vi "CHEM_BOX_TEST_APP.vi"() -> ()   [LabVIEW 2011]
uses:
  <vilib>/Instr/_visa.llb/VISA Set IO Buffer Mask.ctl
  <vilib>/Platform/TimedLoop/XDataNode/timing_clust.ctl
  <vilib>/Platform/TimedLoop/XDataNode/nitl_modes.ctl
  <vilib>/Platform/TimedLoop/XDataNode/wakeup.ctl
  <vilib>/Instr/_visa.llb/VISA Configure Serial Port (Instr).vi
  <vilib>/Platform/TimedLoop/XDataNode/XDataNode.xnode
  <vilib>/Platform/TimedLoop/XDataNode/XDNodeRunTimeDep.lvlib
panel:
  out "4 to 20mA Inputs":dbl[](array[numeric]) format="%#5_5g"
  in  "Stream Inputs":bool
  out "Temperature Sensors":dbl[](array[numeric]) format="%#1_2g"
  out "MISC ADC Inputs":dbl[](array[numeric]) format="%#1_3g"
  out "MFC ADC Inputs":dbl[](array[numeric]) format="%#3_3g"
  in  "MFC Power Control":bool
  in  "MISC DAC Outputs":dbl[](array[slide]) scale=0.0..5.0
  in  "MFC DAC Outputs":dbl[](array[slide])=[0.0, 0.0, 0.0, 0.0, 0.0, 0.0, 0.0] scale=0.0..5.0
  in  "Misc Digital Outputs":bool[](array[boolean])=[FALSE, FALSE, FALSE, FALSE]
  in  "Solenoid Channels":bool[](array[boolean])=[FALSE, FALSE, FALSE, FALSE, FALSE, FALSE, FALSE, FALSE, FALSE, FALSE, FALSE, FALSE]
  in  "FAN CONTROL":bool
  in  "Disable All Heaters and Solenoids":bool
  out "Output Commands":string
  in  "Heater Channels":bool[](array[boolean])=[FALSE, FALSE, FALSE, FALSE, FALSE, FALSE, FALSE, FALSE]
  in  "COM PORT":refnum<visa-resource-name>
  out "Output Command Queue":refnum<queue>
  in  "?":bool
  out "Input Command Queue":refnum<queue>
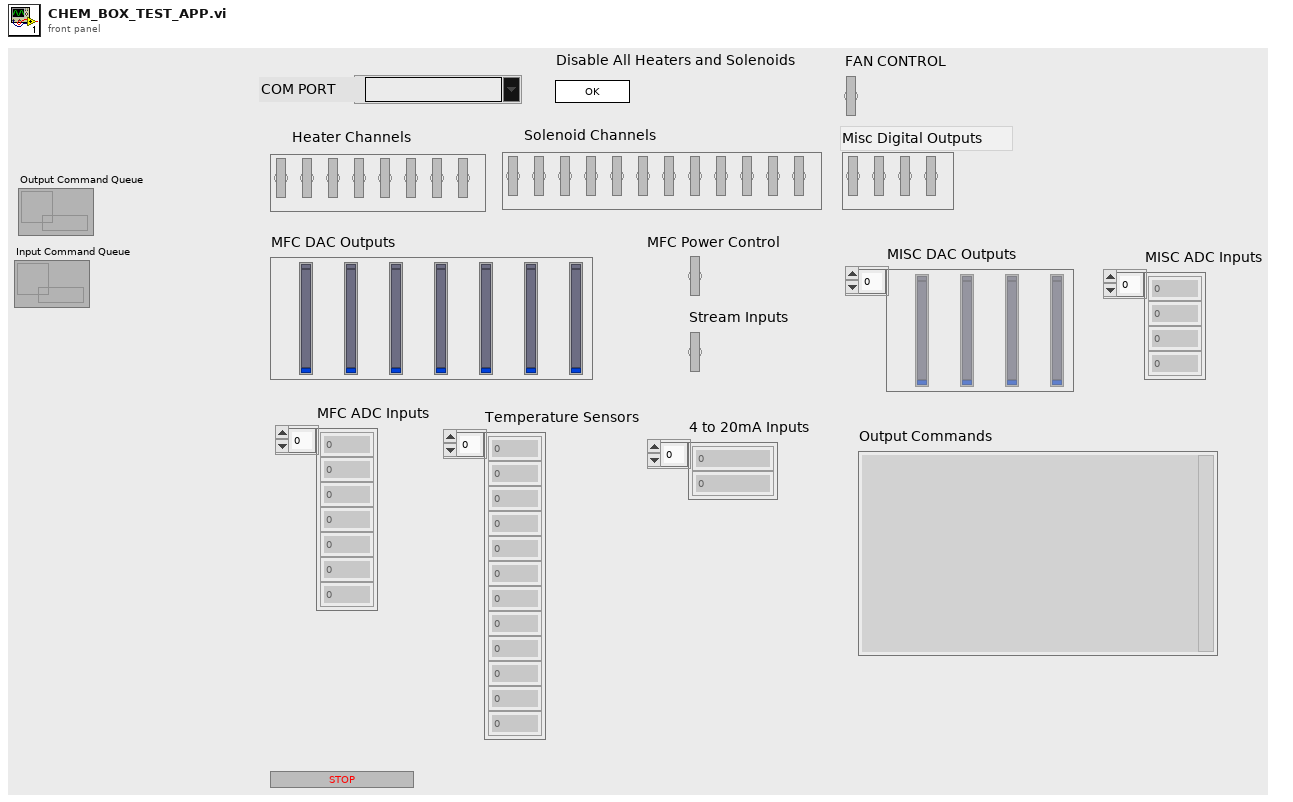
[diagram p1: front panel]
types:
  T1 = typedef "XDNodeRunTimeDep.lvlib/timing_clust.ctl" = cluster{"Expected End [f-1]":u64, "Actual End [f-1]":u64, "Finished Late? [f-1]":bool, "Expected End [i-1]":u64, "Actual End [i-1]":u64, "Finished Late? [i-1]":bool, "Expected Start [i]":u64, "Actual Start [i]":u64, "Expected Start [f]":u64, "Actual Start [f]":u64, "Source Name":string, "Structure Name":string, "Period":i64, "Deadline":i64, "Offset":i64, "Start":i64, "Priority":i32, "Timeout":i32, "Mode":T2, "Wakeup Reason":T3, "Error":errorcluster, "Source Type":string, "Secondary Source Type":string, "Global End Time":u64, "Global Start Time":u64, "Frame Duration":u64, "Iteration Duration":u64, "Assigned CPU":i32, "I/O Scan Engine Mode":u32}
  T2 = typedef "XDNodeRunTimeDep.lvlib/nitl_modes.ctl" = enum32{"No Change", "Process missed periods, maintain original phase", "Discard missed periods, maintain original phase", "Process missed periods, ignore original phase", "Discard missed periods, ignore original phase"}
  T3 = typedef "XDNodeRunTimeDep.lvlib/wakeup.ctl" = enum32{"Normal", "Aborted", "Asynchronous wakeup", "Timing source error", "Timed loop error", "Timeout"}
  T4 = typedef "VISA Set IO Buffer Mask.ctl" = u16
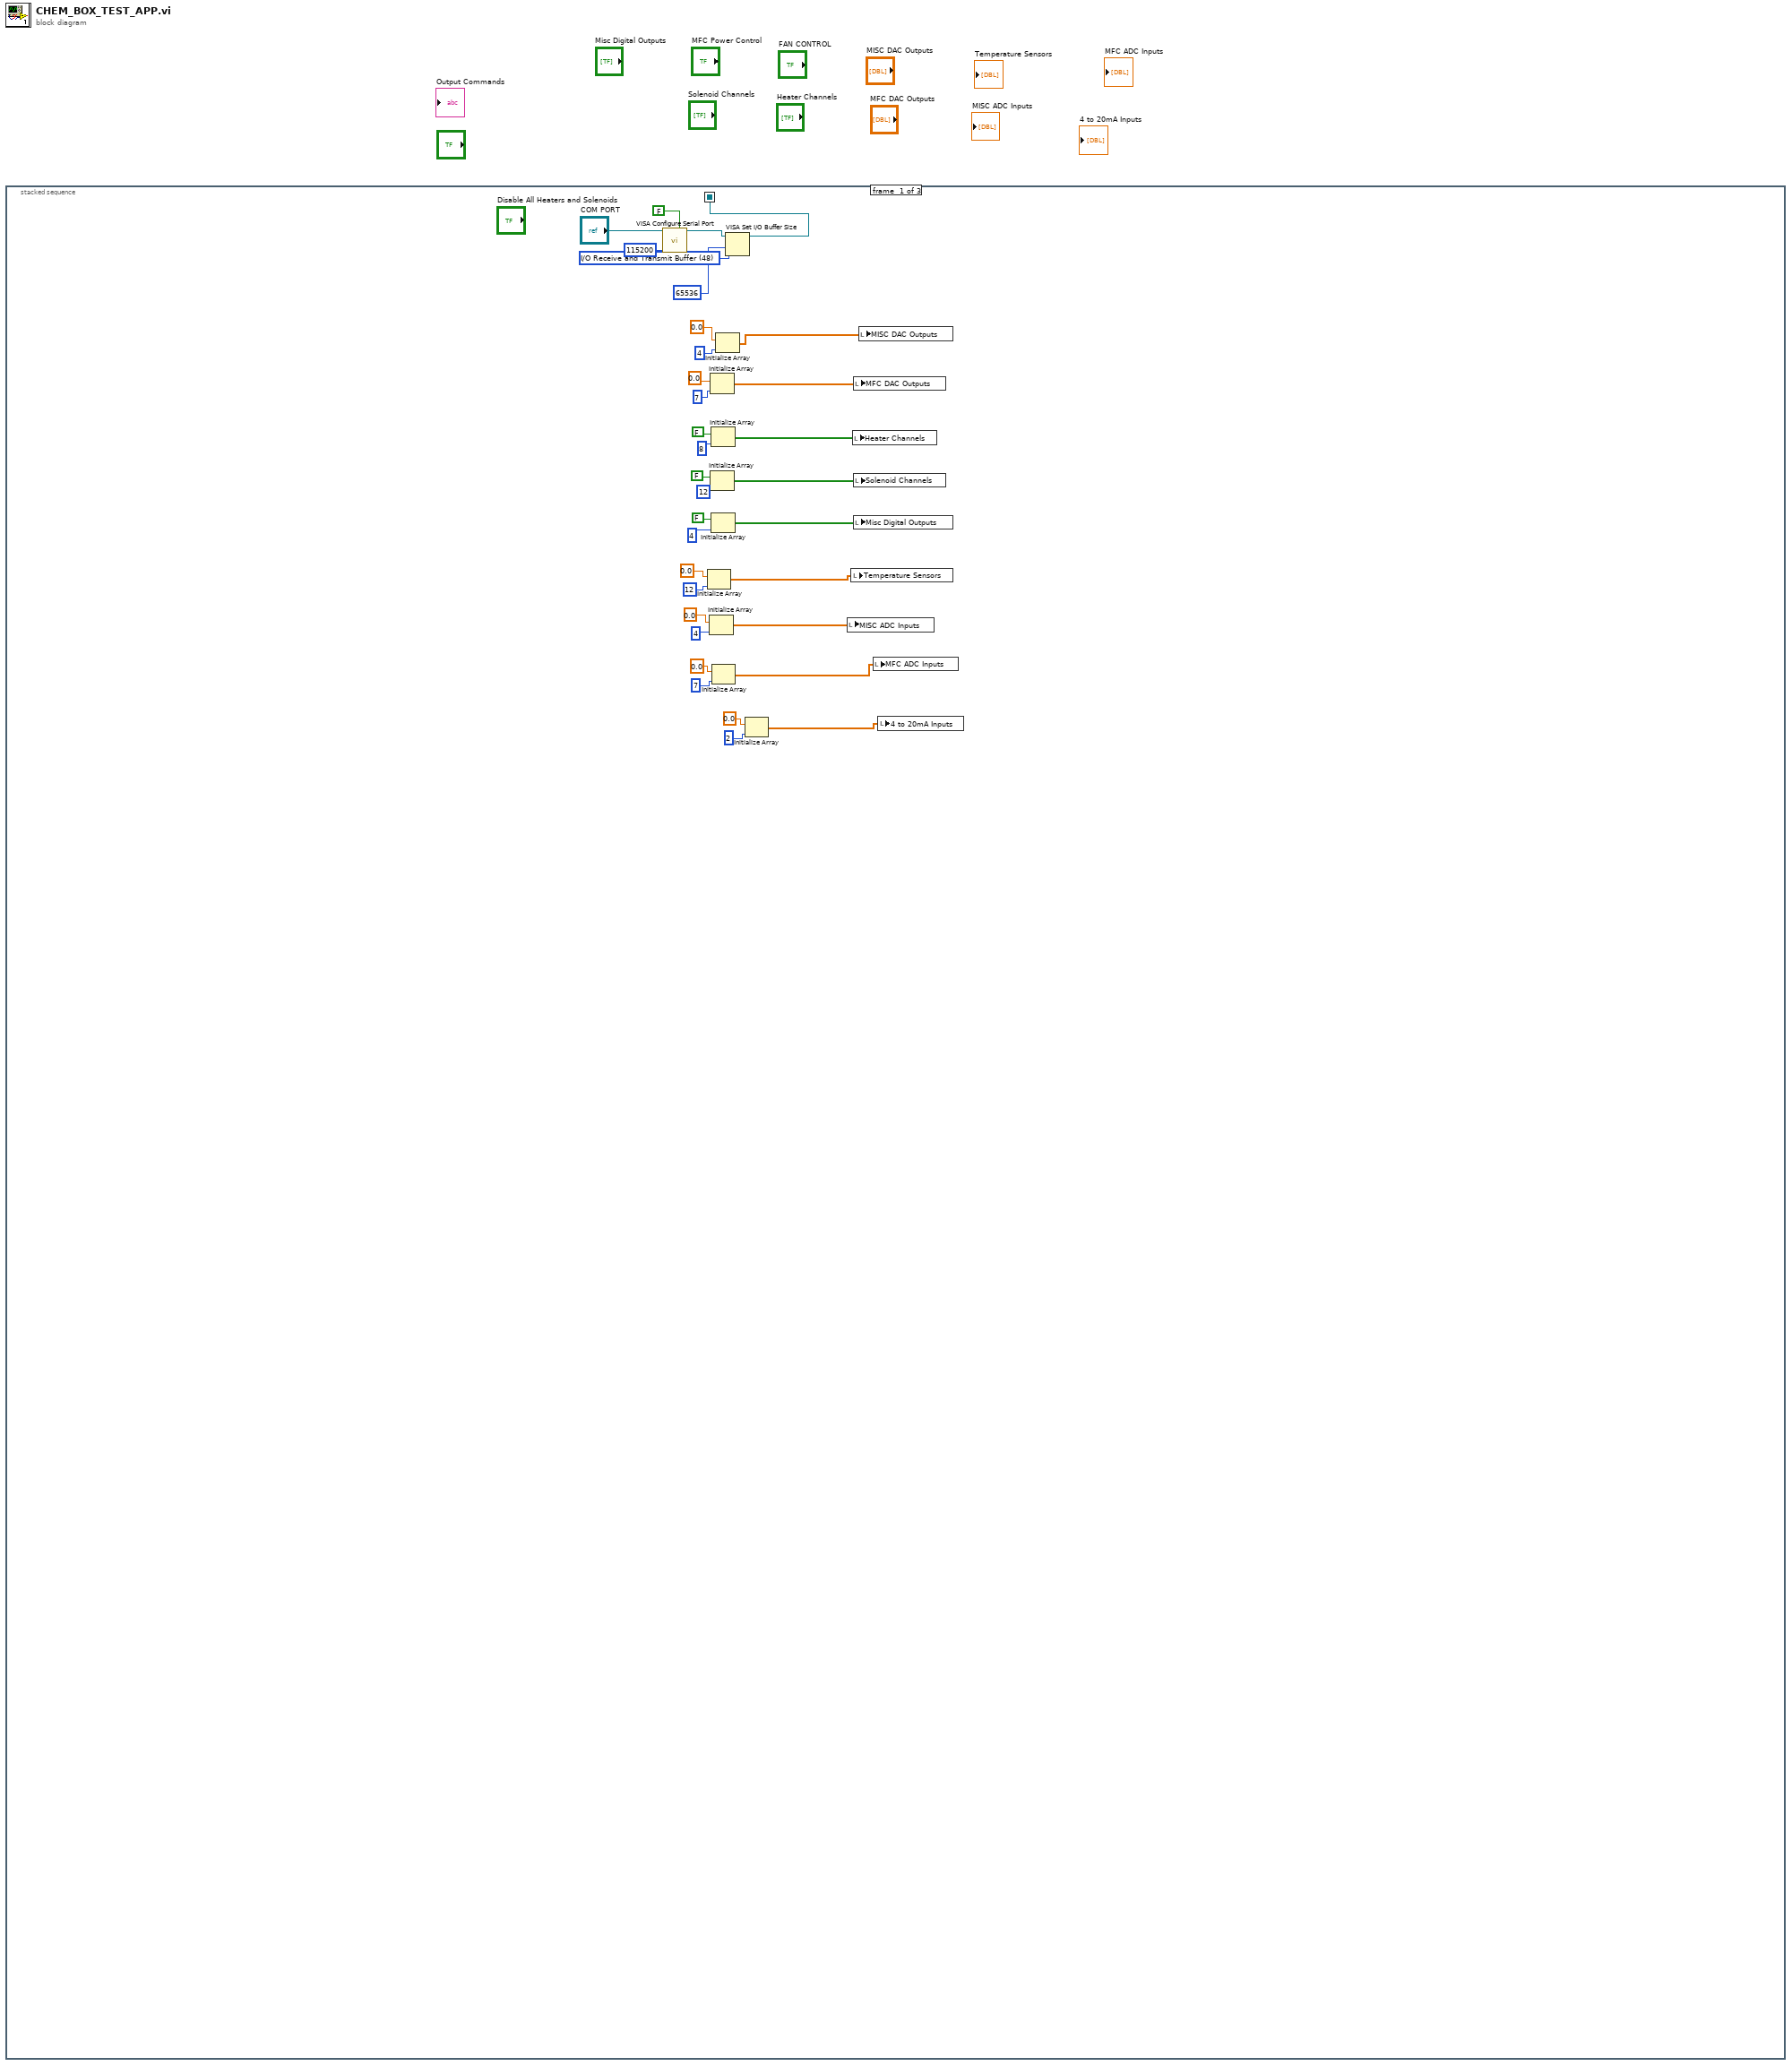
[diagram p0: block diagram]
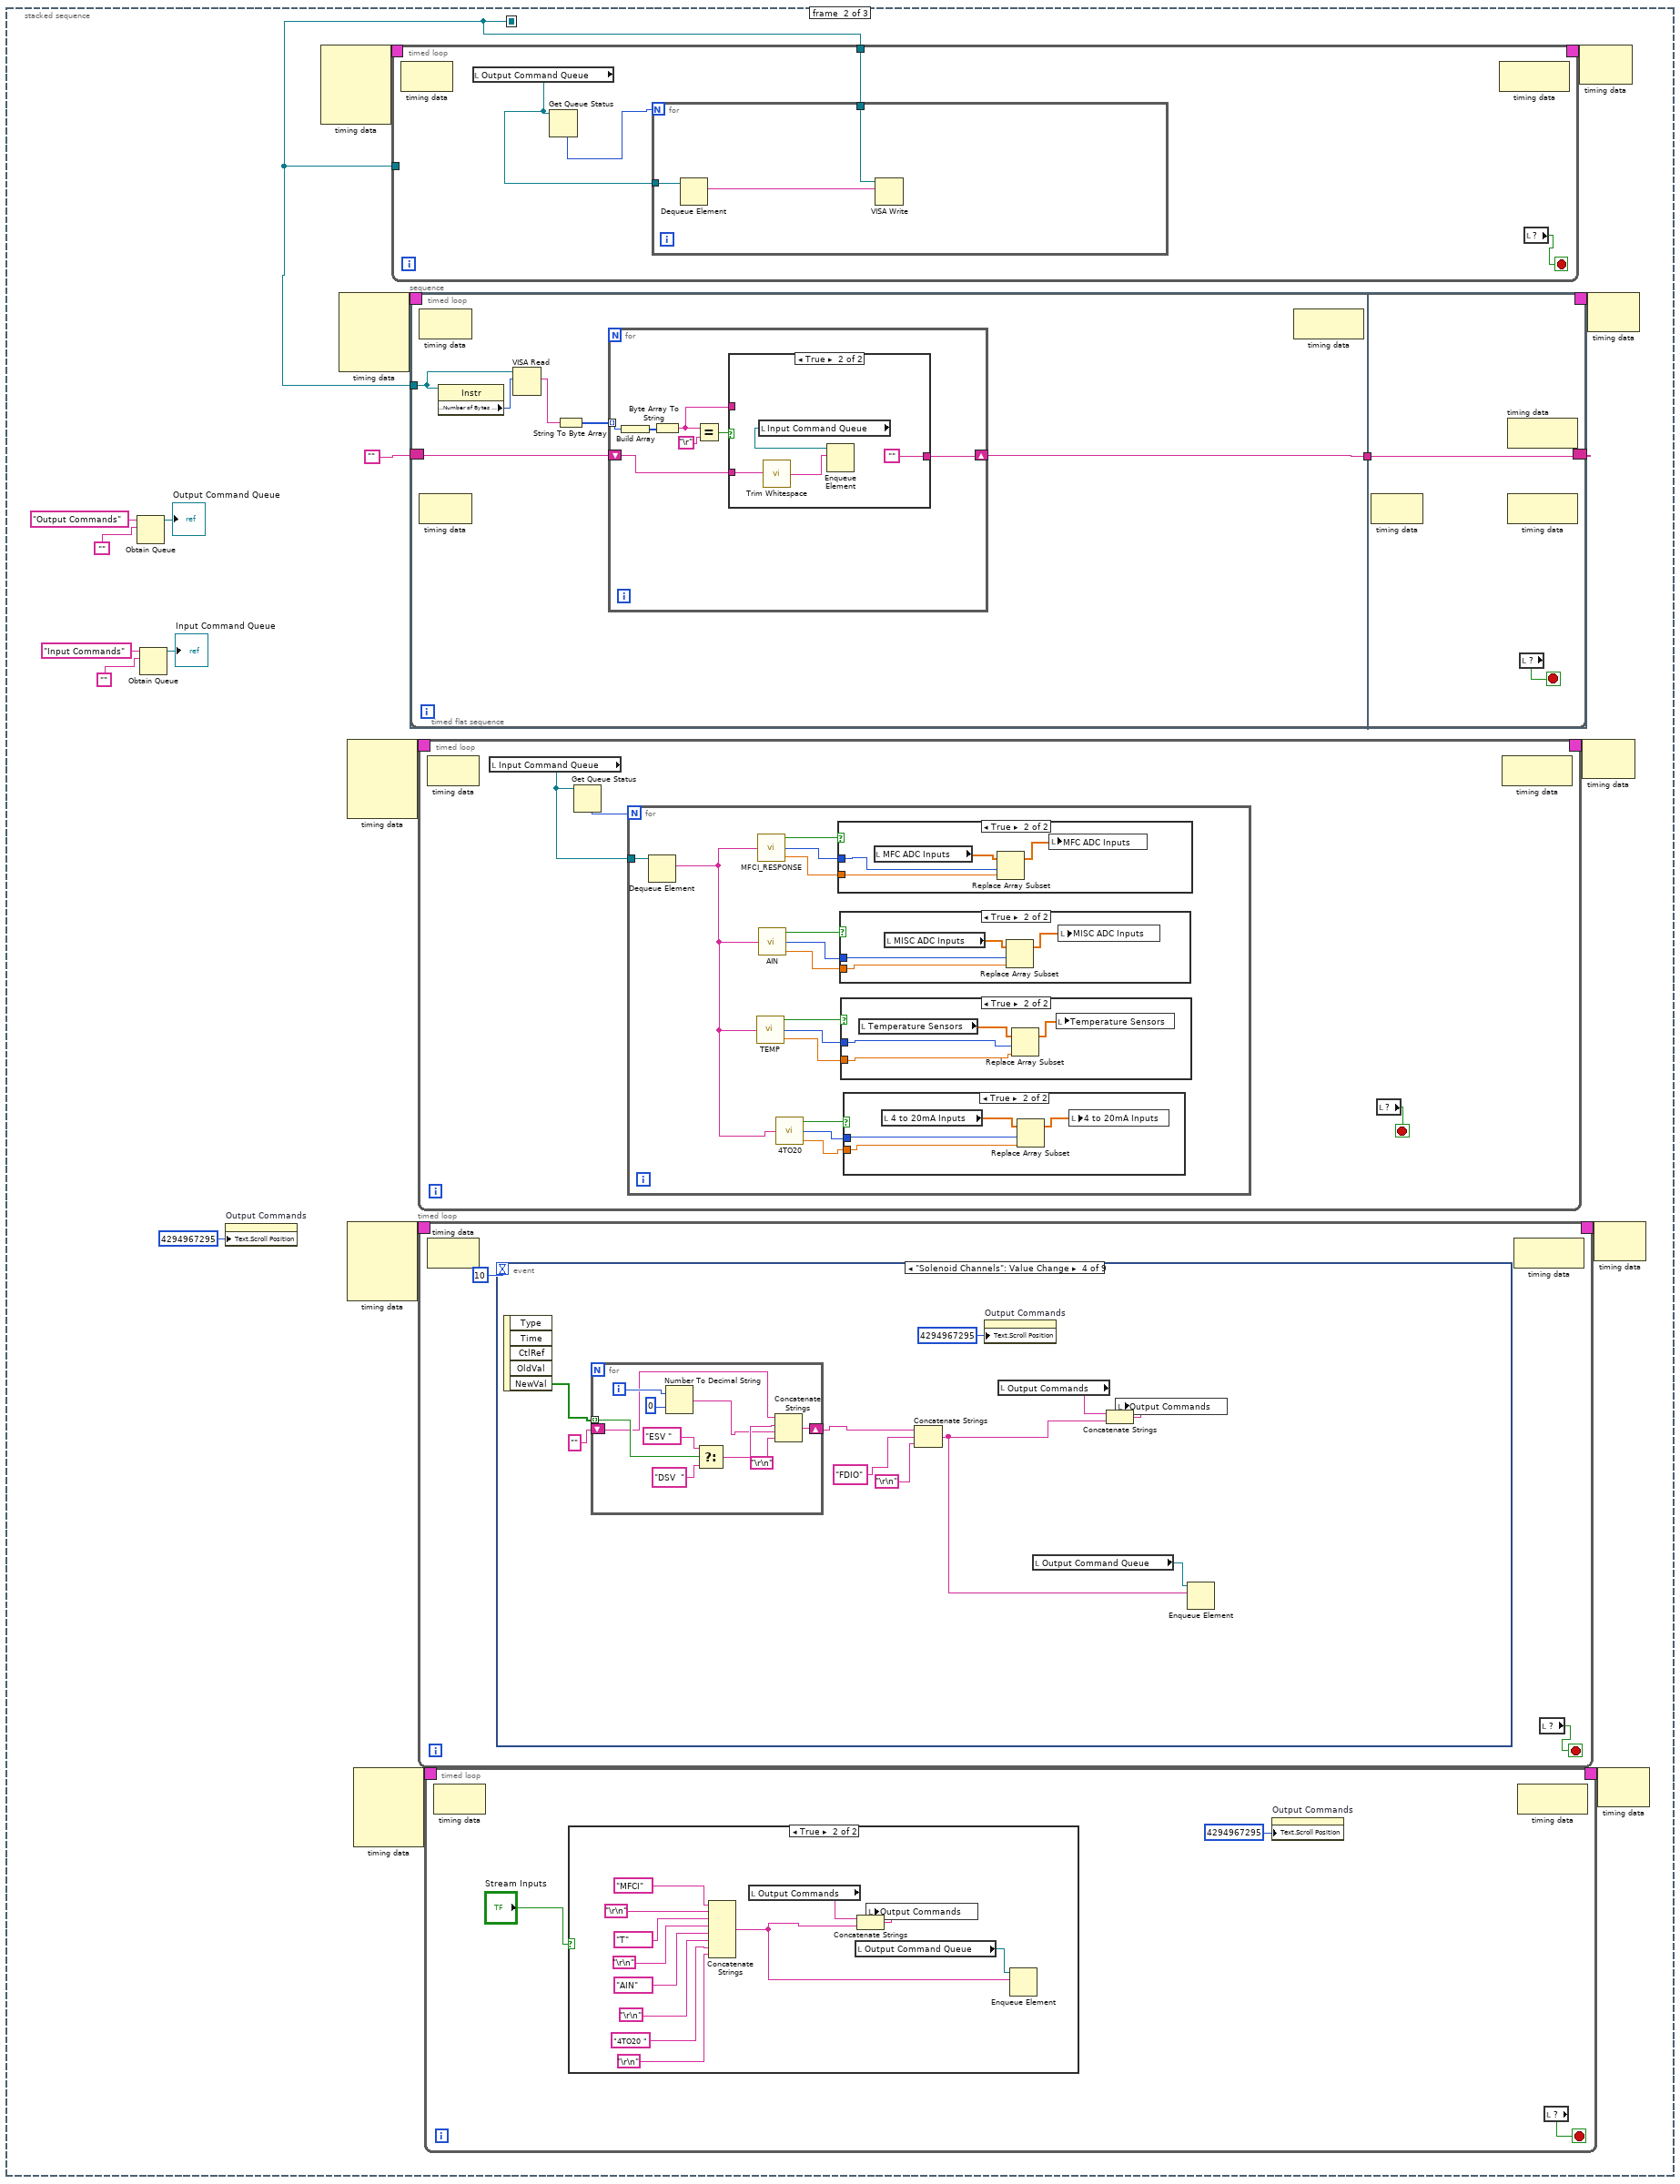
[diagram p2: hidden frame]
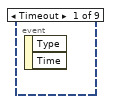
[diagram p4: hidden frame]
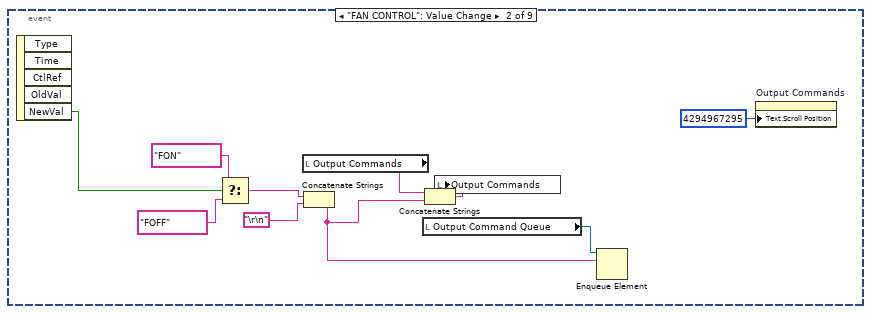
[diagram p5: hidden frame]
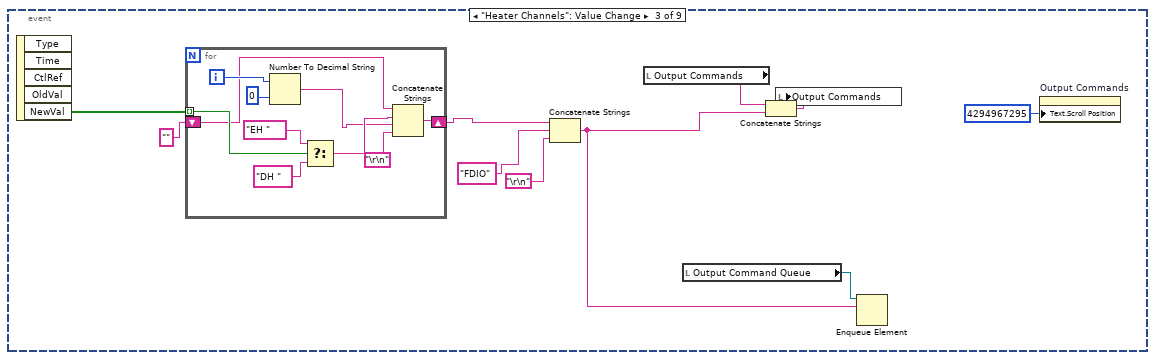
[diagram p6: hidden frame]
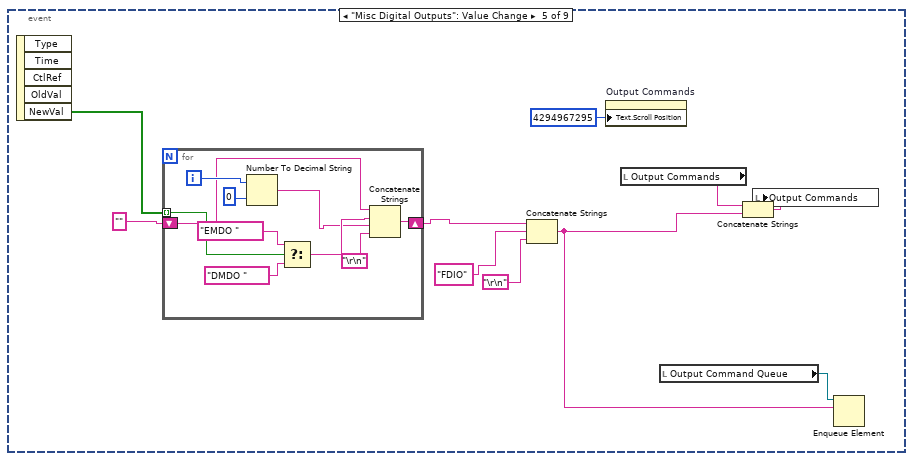
[diagram p7: hidden frame]
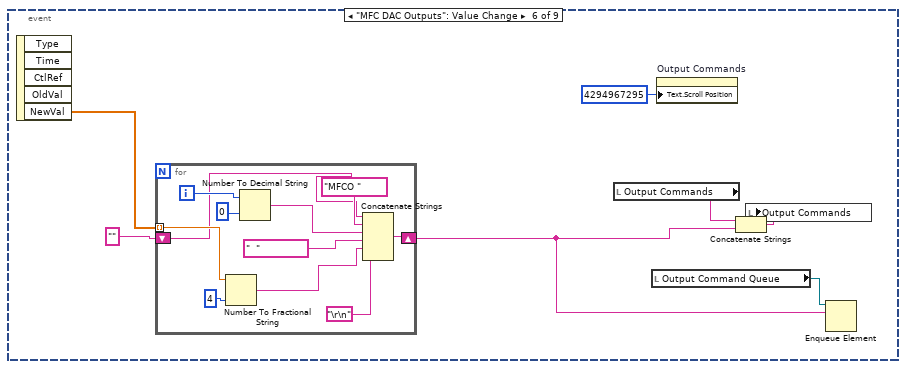
[diagram p8: hidden frame]
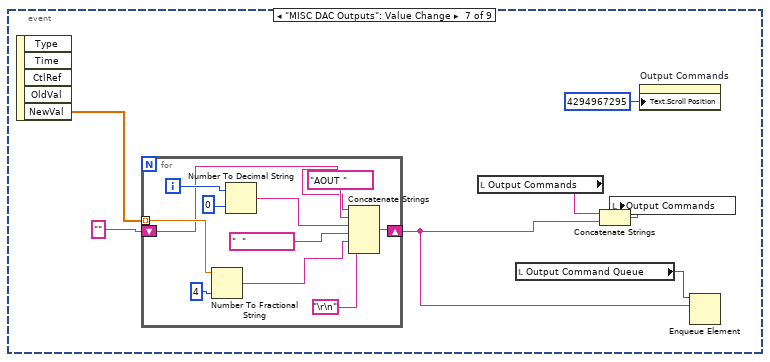
[diagram p9: hidden frame]
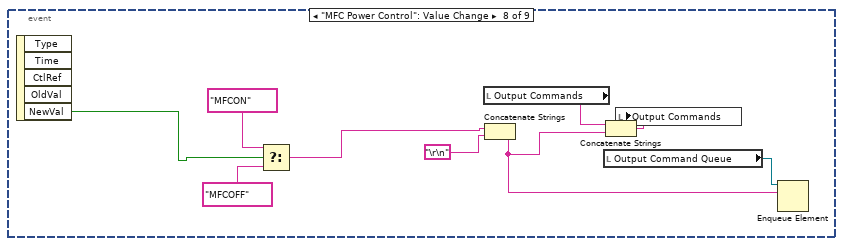
[diagram p10: hidden frame]
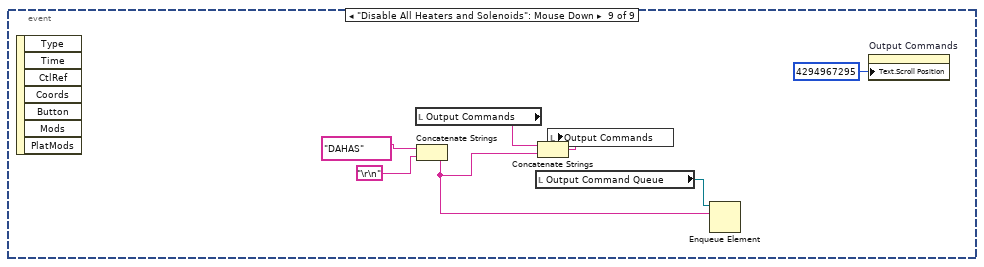
[diagram p11: hidden frame]
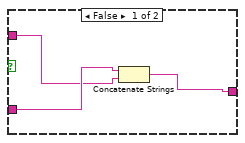
[diagram p16: hidden frame]
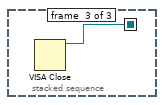
[diagram p17: hidden frame]
diagram:
  n1 = stacked-sequence {
    seq-local: [w30 _ _] -> [_ w40 w287]
    frame #0 {
      w28 = T4 48 items=["I/O Receive Buffer"=16, "I/O Transmit Buffer"=32, "I/O Receive and Transmit Buffer"=48] ("Mask")
      n2 = call-poly "VISA Configure Serial Port"("VISA resource name"="COM PORT", "Enable Termination\nChar (T)"=FALSE ("Enable Termination\nChar (T)"), "baud rate (9600)"=u32 115200) -> ("VISA resource name out"=w31:refnum<visa-resource-name>)  [unwired: 11 in, 1 out]
      n3 = Initialize Array(0.0, 12) -> (w4:dbl[])
      n4 = Initialize Array(0.0, 4) -> (w5:dbl[])
      n5 = Initialize Array(0.0, 7) -> (w17:dbl[])
      n6 = Initialize Array(FALSE, 12) -> (w22:bool[])
      n7 = Initialize Array(FALSE, 8) -> (w25:bool[])
      n8 = Initialize Array(FALSE, 4) -> (w19:bool[])
      n9 = Initialize Array(0.0, 7) -> (w6:dbl[])
      n10 = Initialize Array(0.0, 4) -> (w15:dbl[])
      n11 = VISA Set I/O Buffer Size(VISA resource name=w31, mask (16)=w28, size (4096)=u32 65536) -> (VISA resource name out=w30:refnum<visa-resource-name>)  [unwired: 1 in, 1 out]
      n12 = Initialize Array(0.0, 2) -> (w1:dbl[])
      n13 = local write "MISC ADC Inputs"(w5) -> ()
      n14 = local write "Temperature Sensors"(w4) -> ()
      n15 = local write "Heater Channels"(w25) -> ()
      n16 = local write "MFC DAC Outputs"(w17) -> ()
      n17 = local write "Solenoid Channels"(w22) -> ()
      n18 = local write "Misc Digital Outputs"(w19) -> ()
      n19 = local write "MISC DAC Outputs"(w15) -> ()
      n20 = local write "MFC ADC Inputs"(w6) -> ()
      n21 = local write "4 to 20mA Inputs"(w1) -> ()
    }
    frame #1 {
      n22 = Obtain Queue(name (unnamed)="Output Commands", element data type="") -> (queue out=→"Output Command Queue":refnum<queue>)  [unwired: 3 in, 2 out]
      n23 = Obtain Queue(name (unnamed)="Input Commands", element data type="") -> (queue out=→"Input Command Queue":refnum<queue>)  [unwired: 3 in, 2 out]
      n24 = property on="Output Commands" class="Str"("Text.Scroll Position"=u32 4294967295) -> ()  [unwired: 2 in, 2 out]
      n25 = node-c288() -> (w45:T1)  [unwired: 4 in]
      n26 = node-c288() -> (w53:T1)  [unwired: 4 in]
      n27 = node-c288() -> (w51:T1)  [unwired: 4 in]
      n28 = node-c288() -> (w39:T1)  [unwired: 4 in]
      n29 = node-c288() -> (w36:T1)  [unwired: 4 in]
      n30 = timed-loop {
        timing: w45 -> [_]
        timing-out: [_] -> w44
        tunnel: w40 -> [w205]
        tunnel: [w205] -> _
        tunnel: w40 -> [w202]
        stop <- w201 stop-if-true
        n31 = node-c288() -> ()  [unwired: 1 in, 1 out]
        n32 = local read "Output Command Queue"() -> (w203:refnum<queue>)
        n33 = Get Queue Status(queue=w203) -> (# elements in queue=w204:i32)  [unwired: 2 in, 7 out]
        n34 = for {
          N: w204 -> [_]
          tunnel: w203 -> [w208]
          tunnel: w202 -> [w207]
          n35 = Dequeue Element(queue=w208) -> (element=w206:string)  [unwired: 2 in, 3 out]
          n36 = VISA Write(VISA resource name=w207, write buffer=w206) -> ()  [unwired: 1 in, 3 out]
        }
        n37 = node-c288() -> ()  [unwired: 1 in, 1 out]
        n38 = local read item#1() -> (w201:bool)
      }
      n39 = timed-loop {
        timing: w53 -> [_]
        timing-out: [_] -> w52
        shift-right: [w250] -> _
        shift-left: "" -> [w251]
        tunnel: w40 -> [w252]
        stop <- w279 stop-if-true
        n40 = timed-sequence {
          timing: _ -> [_]
          timing-out: _ -> [_]
          tunnel: w252 -> [w256]
          tunnel: w251 -> [w255]
          tunnel: [w254] -> w250
          n41 = timed-flat-sequence {
            tunnel: w256 -> [w259]
            tunnel: w255 -> [w262]
            tunnel: [w260] -> w253
            tunnel: [w280] -> w254
            tunnel: w253 -> [w280]
            frame #0 {
              n42 = node-c288() -> ()  [unwired: 1 in, 1 out]
              n43 = property class="Instr"(reference=w259) -> ("Serial Settings:Number of Bytes at Serial Port"=w258:u32)  [unwired: 1 in, 2 out]
              n44 = VISA Read(VISA resource name=w259, byte count=w258) -> (read buffer=w257:string)  [unwired: 1 in, 3 out]
              n45 = String To Byte Array(string=w257) -> (unsigned byte array=w261:u8[])
              n46 = for {
                tunnel: w261 -> [w264] mode=indexing
                shift-right: [w266] -> w260
                shift-left: w262 -> [w267]
                n47 = Build Array(w264) -> (w263:u8[])
                n48 = Byte Array To String(unsigned byte array=w263) -> (string=w265:string)
                n49 = Equal?(x=w265, y="\r") -> (x = y?=w268:bool)
                n50 = case shown="True" w268 {
                  tunnel: w267 -> [w272 w275]
                  tunnel: [w270 ""] -> w266
                  tunnel: w265 -> [w271 _]
                  frame False {
                    n51 = Concatenate Strings(w272, w271) -> (w270:string)
                  }
                  frame True {
                    n52 = local read "Input Command Queue"() -> (w276:refnum<queue>)
                    n53 = call <vilib>:"Trim Whitespace.vi"("string"=w275) -> ("trimmed string"=w274:string)  [unwired: 1 in]
                    n54 = Enqueue Element(queue=w276, element=w274) -> ()  [unwired: 2 in, 3 out]
                  }
                }
              }
              n55 = node-c288() -> ()  [unwired: 1 in, 1 out]
            }
            frame #1 {
              n56 = node-c288() -> ()  [unwired: 1 in, 1 out]
              n57 = node-c288() -> ()  [unwired: 1 in, 1 out]
              n58 = local read item#1() -> (w279:bool)
            }
          }
        }
        n59 = node-c288() -> ()  [unwired: 1 in, 1 out]
        n60 = node-c288() -> ()  [unwired: 1 in, 1 out]
      }
      n61 = timed-loop {
        timing: w51 -> [_]
        timing-out: [_] -> w50
        stop <- w213 stop-if-true
        n62 = node-c288() -> ()  [unwired: 1 in, 1 out]
        n63 = local read "Input Command Queue"() -> (w214:refnum<queue>)
        n64 = Get Queue Status(queue=w214) -> (# elements in queue=w215:i32)  [unwired: 2 in, 7 out]
        n65 = for {
          N: w215 -> [_]
          tunnel: w214 -> [w229]
          n66 = Dequeue Element(queue=w229) -> (element=w219:string)  [unwired: 2 in, 3 out]
          n67 = call "TEMP.vi"("Input"=w219) -> ("Match?"=w226:bool, "Channel"=w221:i32, "Data"=w220:dbl)
          n68 = call "MFCI_RESPONSE.vi"("Input"=w219) -> ("Match?"=w228:bool, "Channel"=w225:i32, "Data"=w224:dbl)
          n69 = call "AIN.vi"("Input"=w219) -> ("Match?"=w227:bool, "Channel"=w223:i32, "Data"=w222:dbl)
          n70 = call "4TO20.vi"("Input"=w219) -> ("Match?"=w218:bool, "Channel"=w217:i32, "Data"=w216:dbl)
          n71 = case shown="True" w228 {
            tunnel: w225 -> [_ w243]
            tunnel: w224 -> [_ w242]
            frame False {
            }
            frame True {
              n72 = local read "MFC ADC Inputs"() -> (w244:dbl[])
              n73 = Replace Array Subset(array=w244, new element=w242, index=w243) -> (w245:dbl[])
              n74 = local write "MFC ADC Inputs"(w245) -> ()
            }
          }
          n75 = case shown="True" w227 {
            tunnel: w223 -> [_ w239]
            tunnel: w222 -> [_ w238]
            frame False {
            }
            frame True {
              n76 = local read "MISC ADC Inputs"() -> (w241:dbl[])
              n77 = Replace Array Subset(array=w241, new element=w238, index=w239) -> (w240:dbl[])
              n78 = local write "MISC ADC Inputs"(w240) -> ()
            }
          }
          n79 = case shown="True" w226 {
            tunnel: w221 -> [_ w235]
            tunnel: w220 -> [_ w234]
            frame False {
            }
            frame True {
              n80 = local read "Temperature Sensors"() -> (w236:dbl[])
              n81 = Replace Array Subset(array=w236, new element=w234, index=w235) -> (w237:dbl[])
              n82 = local write "Temperature Sensors"(w237) -> ()
            }
          }
          n83 = case shown="True" w218 {
            tunnel: w217 -> [_ w232]
            tunnel: w216 -> [_ w231]
            frame False {
            }
            frame True {
              n84 = local read "4 to 20mA Inputs"() -> (w233:dbl[])
              n85 = Replace Array Subset(array=w233, new element=w231, index=w232) -> (w230:dbl[])
              n86 = local write "4 to 20mA Inputs"(w230) -> ()
            }
          }
        }
        n87 = local read item#1() -> (w213:bool)
        n88 = node-c288() -> ()  [unwired: 1 in, 1 out]
      }
      n89 = timed-loop {
        timing: w39 -> [_]
        timing-out: [_] -> w38
        stop <- w73 stop-if-true
        n90 = node-c288() -> ()  [unwired: 1 in, 1 out]
        n91 = event shown="[3] \"Solenoid Channels\": Value Change" {
          selector: _ -> [_ _ _ _ _ _ _ _ _]
          dyn-events: _ -> [_ _ _ _ _ _ _ _ _]
          timeout: 10 -> [_ _ _ _ _ _ _ _ _]
          event Timeout {
            n92 = event-data() -> ()  [unwired: 1 in, 2 out]
          }
          event "FAN CONTROL": Value Change {
            n93 = event-data() -> ("NewVal"=w75:bool)  [unwired: 1 in, 4 out]
            n94 = Select(t="FON", s=w75, f="FOFF") -> (s? t:f=w78:string)
            n95 = local read "Output Commands"() -> (w83:string)
            n96 = Concatenate Strings(w78, "\r\n") -> (w80:string)
            n97 = local read "Output Command Queue"() -> (w81:refnum<queue>)
            n98 = Concatenate Strings(w83, w80) -> (w82:string)
            n99 = local write "Output Commands"(w82) -> ()
            n100 = Enqueue Element(queue=w81, element=w80) -> ()  [unwired: 2 in, 3 out]
            n101 = property on="Output Commands" class="Str"("Text.Scroll Position"=u32 4294967295) -> ()  [unwired: 2 in, 2 out]
          }
          event "Heater Channels": Value Change {
            n102 = event-data() -> ("NewVal"=w94:bool[])  [unwired: 1 in, 4 out]
            n103 = for {
              tunnel: w94 -> [w102] mode=indexing
              shift-right: [w95] -> w92
              shift-left: "" -> [w96]
              i -> [w104]
              n104 = Number To Decimal String(number=w104, width (-)=0) -> (decimal integer string=w98:string)
              n105 = Select(t="EH ", s=w102, f="DH ") -> (s? t:f=w99:string)
              n106 = Concatenate Strings(w96, w99, w98, "\r\n") -> (w95:string)
            }
            n107 = Concatenate Strings(w92, "FDIO", "\r\n") -> (w86:string)
            n108 = local read "Output Commands"() -> (w89:string)
            n109 = local read "Output Command Queue"() -> (w87:refnum<queue>)
            n110 = Concatenate Strings(w89, w86) -> (w88:string)
            n111 = local write "Output Commands"(w88) -> ()
            n112 = Enqueue Element(queue=w87, element=w86) -> ()  [unwired: 2 in, 3 out]
            n113 = property on="Output Commands" class="Str"("Text.Scroll Position"=u32 4294967295) -> ()  [unwired: 2 in, 2 out]
          }
          event "Solenoid Channels": Value Change {
            n114 = event-data() -> ("NewVal"=w105:bool[])  [unwired: 1 in, 4 out]
            n115 = for {
              tunnel: w105 -> [w122] mode=indexing
              shift-right: [w115] -> w113
              shift-left: "" -> [w116]
              i -> [w124]
              n116 = Number To Decimal String(number=w124, width (-)=0) -> (decimal integer string=w118:string)
              n117 = Select(t="ESV ", s=w122, f="DSV  ") -> (s? t:f=w119:string)
              n118 = Concatenate Strings(w116, w119, w118, "\r\n") -> (w115:string)
            }
            n119 = Concatenate Strings(w113, "FDIO", "\r\n") -> (w107:string)
            n120 = property on="Output Commands" class="Str"("Text.Scroll Position"=u32 4294967295) -> ()  [unwired: 2 in, 2 out]
            n121 = local read "Output Commands"() -> (w110:string)
            n122 = local read "Output Command Queue"() -> (w108:refnum<queue>)
            n123 = Concatenate Strings(w110, w107) -> (w109:string)
            n124 = local write "Output Commands"(w109) -> ()
            n125 = Enqueue Element(queue=w108, element=w107) -> ()  [unwired: 2 in, 3 out]
          }
          event "Misc Digital Outputs": Value Change {
            n126 = event-data() -> ("NewVal"=w125:bool[])  [unwired: 1 in, 4 out]
            n127 = for {
              tunnel: w125 -> [w142] mode=indexing
              shift-right: [w135] -> w133
              shift-left: "" -> [w136]
              i -> [w144]
              n128 = Number To Decimal String(number=w144, width (-)=0) -> (decimal integer string=w138:string)
              n129 = Select(t="EMDO ", s=w142, f="DMDO ") -> (s? t:f=w139:string)
              n130 = Concatenate Strings(w136, w139, w138, "\r\n") -> (w135:string)
            }
            n131 = Concatenate Strings(w133, "FDIO", "\r\n") -> (w127:string)
            n132 = property on="Output Commands" class="Str"("Text.Scroll Position"=u32 4294967295) -> ()  [unwired: 2 in, 2 out]
            n133 = local read "Output Commands"() -> (w130:string)
            n134 = local read "Output Command Queue"() -> (w128:refnum<queue>)
            n135 = Concatenate Strings(w130, w127) -> (w129:string)
            n136 = local write "Output Commands"(w129) -> ()
            n137 = Enqueue Element(queue=w128, element=w127) -> ()  [unwired: 2 in, 3 out]
          }
          event "MFC DAC Outputs": Value Change {
            n138 = event-data() -> ("NewVal"=w147:dbl[])  [unwired: 1 in, 4 out]
            n139 = for {
              tunnel: w147 -> [w154] mode=indexing
              shift-right: [w160] -> w146
              shift-left: "" -> [w152]
              i -> [w162]
              n140 = Number To Fractional String(number=w154, precision (6)=i16 4 ("width (-)")) -> (F-format string=w156:string)  [unwired: 2 in]
              n141 = Number To Decimal String(number=w162, width (-)=0) -> (decimal integer string=w159:string)
              n142 = Concatenate Strings(w152, "MFCO ", w159, "  ", w156, "\r\n") -> (w160:string)
            }
            n143 = local read "Output Commands"() -> (w150:string)
            n144 = local read "Output Command Queue"() -> (w148:refnum<queue>)
            n145 = property on="Output Commands" class="Str"("Text.Scroll Position"=u32 4294967295) -> ()  [unwired: 2 in, 2 out]
            n146 = Concatenate Strings(w150, w146) -> (w149:string)
            n147 = local write "Output Commands"(w149) -> ()
            n148 = Enqueue Element(queue=w148, element=w146) -> ()  [unwired: 2 in, 3 out]
          }
          event "MISC DAC Outputs": Value Change {
            n149 = event-data() -> ("NewVal"=w164:dbl[])  [unwired: 1 in, 4 out]
            n150 = for {
              tunnel: w164 -> [w172] mode=indexing
              shift-right: [w178] -> w165
              shift-left: "" -> [w170]
              i -> [w180]
              n151 = Number To Fractional String(number=w172, precision (6)=i16 4 ("width (-)")) -> (F-format string=w174:string)  [unwired: 2 in]
              n152 = Number To Decimal String(number=w180, width (-)=0) -> (decimal integer string=w177:string)
              n153 = Concatenate Strings(w170, "AOUT ", w177, "  ", w174, "\r\n") -> (w178:string)
            }
            n154 = local read "Output Commands"() -> (w168:string)
            n155 = local read "Output Command Queue"() -> (w166:refnum<queue>)
            n156 = Concatenate Strings(w168, w165) -> (w167:string)
            n157 = local write "Output Commands"(w167) -> ()
            n158 = property on="Output Commands" class="Str"("Text.Scroll Position"=u32 4294967295) -> ()  [unwired: 2 in, 2 out]
            n159 = Enqueue Element(queue=w166, element=w165) -> ()  [unwired: 2 in, 3 out]
          }
          event "MFC Power Control": Value Change {
            n160 = event-data() -> ("NewVal"=w189:bool)  [unwired: 1 in, 4 out]
            n161 = Select(t="MFCON", s=w189, f="MFCOFF") -> (s? t:f=w183:string)
            n162 = local read "Output Commands"() -> (w187:string)
            n163 = Concatenate Strings(w183, "\r\n") -> (w184:string)
            n164 = local read "Output Command Queue"() -> (w185:refnum<queue>)
            n165 = Concatenate Strings(w187, w184) -> (w186:string)
            n166 = local write "Output Commands"(w186) -> ()
            n167 = Enqueue Element(queue=w185, element=w184) -> ()  [unwired: 2 in, 3 out]
          }
          event "Disable All Heaters and Solenoids": Mouse Down {
            n168 = event-data() -> ()  [unwired: 1 in, 7 out]
            n169 = local read "Output Commands"() -> (w194:string)
            n170 = Concatenate Strings("DAHAS", "\r\n") -> (w191:string)
            n171 = local read "Output Command Queue"() -> (w192:refnum<queue>)
            n172 = Concatenate Strings(w194, w191) -> (w193:string)
            n173 = local write "Output Commands"(w193) -> ()
            n174 = Enqueue Element(queue=w192, element=w191) -> ()  [unwired: 2 in, 3 out]
            n175 = property on="Output Commands" class="Str"("Text.Scroll Position"=u32 4294967295) -> ()  [unwired: 2 in, 2 out]
          }
        }
        n176 = node-c288() -> ()  [unwired: 1 in, 1 out]
        n177 = local read item#1() -> (w73:bool)
      }
      n178 = timed-loop {
        timing: w36 -> [_]
        timing-out: [_] -> w35
        stop <- w56 stop-if-true
        n179 = node-c288() -> ()  [unwired: 1 in, 1 out]
        n180 = case shown="True" "Stream Inputs" {
          frame False {
          }
          frame True {
            n181 = Concatenate Strings("MFCI", "\r\n", "T", "\r\n", "AIN", "\r\n", "4TO20 ", "\r\n") -> (w65:string)
            n182 = local read "Output Commands"() -> (w68:string)
            n183 = local read "Output Command Queue"() -> (w66:refnum<queue>)
            n184 = Concatenate Strings(w68, w65) -> (w67:string)
            n185 = local write "Output Commands"(w67) -> ()
            n186 = Enqueue Element(queue=w66, element=w65) -> ()  [unwired: 2 in, 3 out]
          }
        }
        n187 = property on="Output Commands" class="Str"("Text.Scroll Position"=u32 4294967295) -> ()  [unwired: 2 in, 2 out]
        n188 = node-c288() -> ()  [unwired: 1 in, 1 out]
        n189 = local read item#1() -> (w56:bool)
      }
      n190 = node-c288(w44) -> ()  [unwired: 1 out]
      n191 = node-c288(w50) -> ()  [unwired: 1 out]
      n192 = node-c288(w52) -> ()  [unwired: 1 out]
      n193 = node-c288(w38) -> ()  [unwired: 1 out]
      n194 = node-c288(w35) -> ()  [unwired: 1 out]
    }
    frame #2 {
      n195 = VISA Close(VISA resource name=w287) -> ()  [unwired: 1 in, 1 out]
    }
  }
